vi "AWS-S3-ListBuckets.vi"(0 "AWS-S3-API":refnum<class "AWS-S3-API.lvclass">, 11 "error in":errorcluster) -> (4 "AWS-S3-API out":refnum<class "AWS-S3-API.lvclass">, 6 "Buckets":string[](array[string]), 15 "error out":errorcluster)   [LabVIEW 2012, in "AWS-S3-API.lvclass"]
uses:
  AWS-S3-API.lvclass
  C:/Users/Jack/repo/aws/AWS-SDK/AWSSDK.dll
  repo/aws/AWS-SDK/AWSSDK.dll
panel:
  # "Inputs"
  # "Outputs"
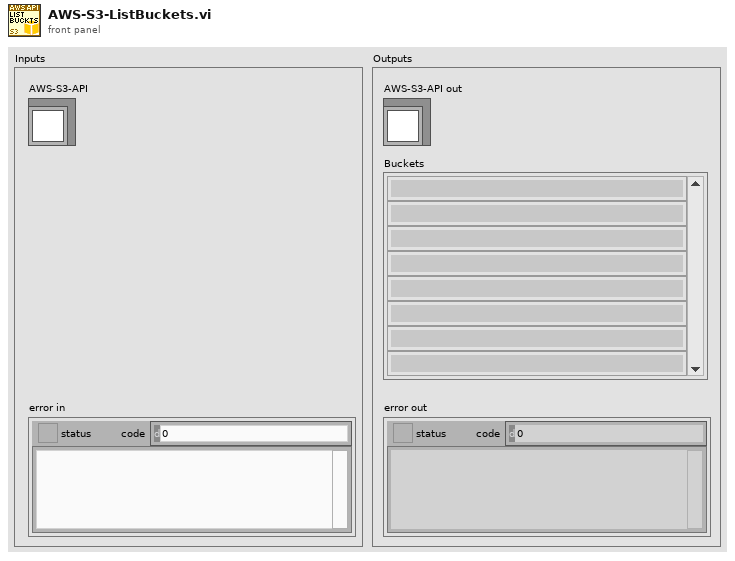
[diagram p1: front panel]
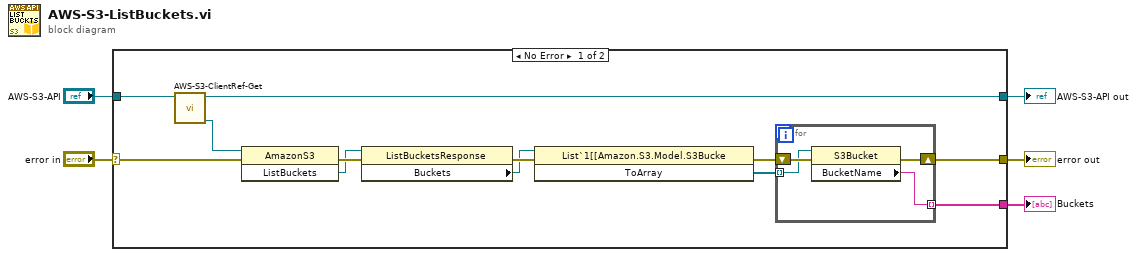
[diagram p0: block diagram]
diagram:
  n1 = case shown="No Error" "error in" {
    selector: "error in" -> [w17 w23]
    tunnel: [w11 w23] -> w5
    tunnel: [w7 w22] -> w3
    tunnel: "AWS-S3-API" -> [w8 w22]
    tunnel: [w12 _] -> w1
    frame No Error {
      n2 = call "AWS-S3-ClientRef-Get.vi"("AWS-S3-API"=w8) -> ("S3 Client ref"=w6:refnum<k24>, "AWS-S3-API out"=w7:refnum<class "AWS-S3-API.lvclass">)  [unwired: 9 in]
      n3 = invoke class="AmazonS3" method="ListBuckets"(reference=w6, error in=w17) -> (error out=w16:errorcluster, "ListBuckets"=w10:refnum<k24>)  [unwired: 1 in, 1 out]
      n4 = property class="ListBucketsResponse"(reference=w10, error in=w16) -> (error out=w15:errorcluster, "Buckets"=w9:refnum<k24>)  [unwired: 1 out]
      n5 = invoke class="List`1[[Amazon.S3.Model.S3Bucke" method="ToArray"(reference=w9, error in=w15) -> (error out=w14:errorcluster, "ToArray"=w13:refnum<k24>[])  [unwired: 1 in, 1 out]
      n6 = for {
        tunnel: w13 -> [w20] mode=indexing
        tunnel: [w18] -> w12 mode=indexing
        shift-right: [w19] -> w11
        shift-left: w14 -> [w21]
        n7 = property class="S3Bucket"(reference=w20, error in=w21) -> (error out=w19:errorcluster, "BucketName"=w18:string)  [unwired: 1 out]
      }
    }
    frame Error {
    }
  }
  "error out" <- w5
  "AWS-S3-API out" <- w3
  "Buckets" <- w1
